vi "SQL表面型号数据库写入.vi"(0 "ADODB._Connection In":refnum<k7>, 5 "ProductNumber":string, 7 "ProductType":string, 9 "ProssureType":string, 11 "error in (no error)":errorcluster caption="错误输入（无错误）") -> (4 "连接的字符串":string, 6 "ADODB._Connection Out":refnum<k7>, 15 "error out":errorcluster caption="错误输出")   [LabVIEW 2017]
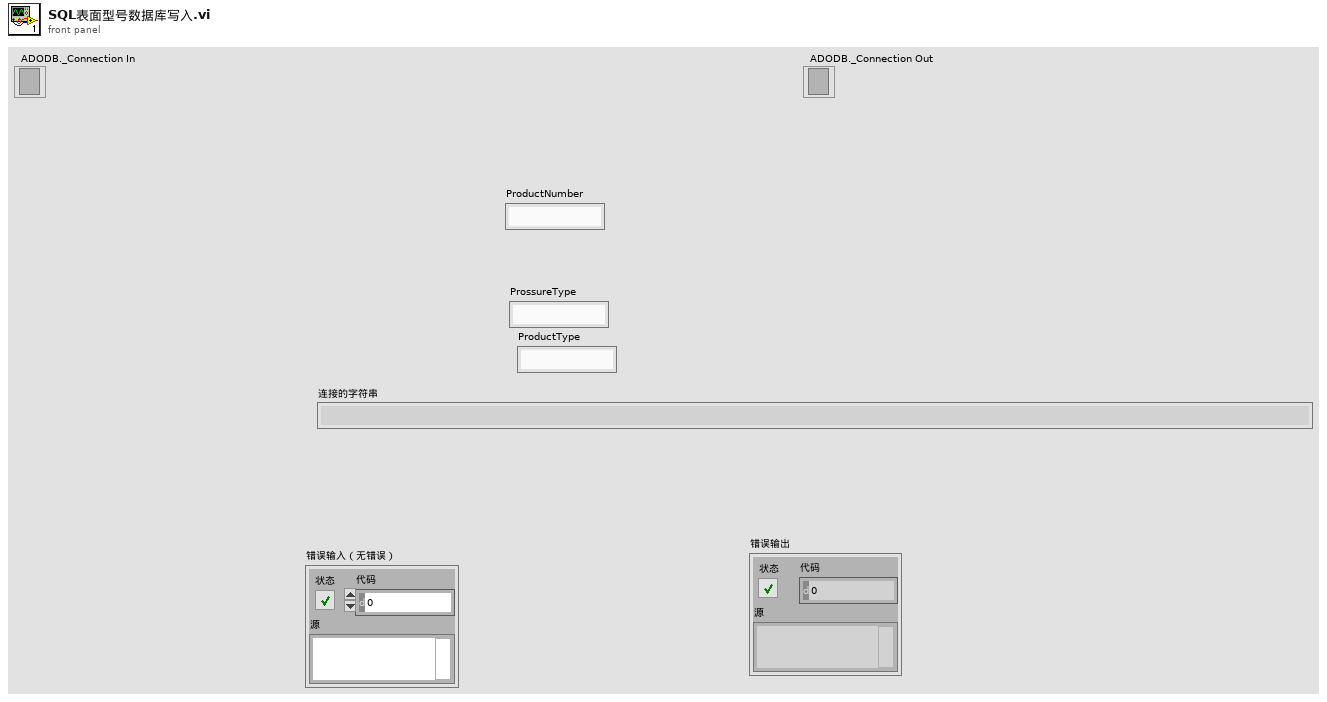
[diagram p1: front panel]
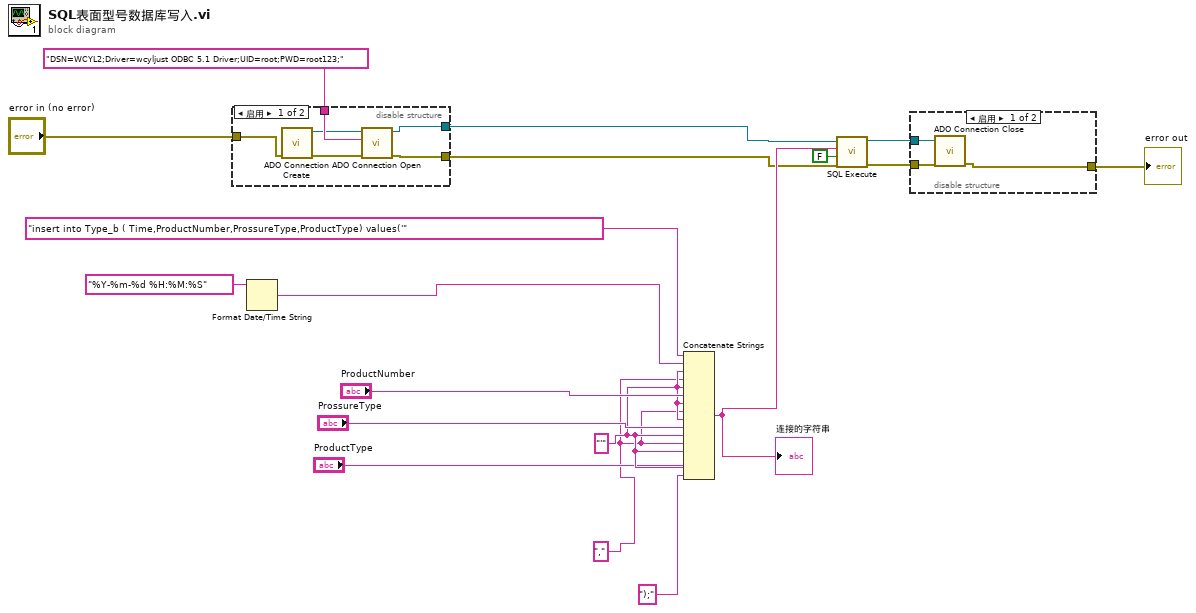
[diagram p0: block diagram]
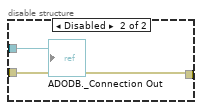
[diagram p2: hidden frame]
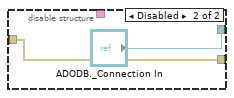
[diagram p3: hidden frame]
diagram:
  w3 = "'" ("字符串")
  w1 = "," ("字符串")
  n1 = disable-structure shown="启用" {
    disable-tunnel: "DSN=WCYL2;Driver=wcyljust ODBC 5.1 Driver;UID=root;PWD=root123;" ("ConnectionString") -> [w24 _]
    disable-tunnel: "error in (no error)" -> [w23 w26]
    disable-tunnel: [w20 "ADODB._Connection In"] -> w5
    disable-tunnel: [w19 w26] -> w4
    frame Enabled {
      n2 = call <userlib>:"ADO Connection Create.vi"("error in (no error)"=w23) -> ("error out"=w21:errorcluster, "ADODB._Connection Out"=w22:refnum<k7>)  [unwired: 9 in]
      n3 = call <userlib>:"ADO Connection Open.vi"("error in (no error)"=w21, "ConnectionString"=w24, "ADODB._Connection In"=w22) -> ("error out"=w19:errorcluster, "ADODB._Connection Out"=w20:refnum<k7>)  [unwired: 7 in]
    }
    frame Disabled {
    }
  }
  n4 = Format Date/Time String(time format string (%c)="%Y-%m-%d %H:%M:%S" ("时间格式字符串(%c)")) -> (date/time string=w10:string)  [unwired: 2 in]
  n5 = Concatenate Strings("insert into Type_b ( Time,ProductNumber,ProssureType,ProductType) values('" ("Command Text"), w10, w3, w1, w3, "ProductNumber", w3, w1, w3, "ProssureType", w3, w1, w3, "ProductType", w3, ");" ("字符串")) -> (w15:string)
  "连接的字符串" <- w15
  n6 = call <userlib>:"SQL Execute.vi"("error in (no error)"=w4, "Return Data (T)"=FALSE, "Command Text"=w15, "ADODB._Connection In"=w5) -> ("error out"=w7:errorcluster, "ADODB._Connection Out"=w8:refnum<k7>)  [unwired: 4 in, 2 out]
  n7 = disable-structure shown="启用" {
    disable-tunnel: [w29 w31] -> w13
    disable-tunnel: w8 -> [w28 w30]
    disable-tunnel: w7 -> [w27 w31]
    frame Enabled {
      n8 = call <userlib>:"ADO Connection Close.vi"("error in (no error)"=w27, "ADODB._Connection In"=w28) -> ("error out"=w29:errorcluster)  [unwired: 8 in, 1 out]
    }
    frame Disabled {
      "ADODB._Connection Out" <- w30
    }
  }
  "error out" <- w13
